vi "Get Publish Data Events.vi"(11 "UserEvents in":refnum<class "User Events.lvclass">) -> (2 "Publish Data Events":T1, 3 "UserEvents out":refnum<class "User Events.lvclass">)   [LabVIEW 2015, in "User Events.lvclass"]
uses:
  User Events.lvclass
  Typedefs/Publish Data Events.ctl
  Typedefs/State Types.ctl
  <userlib>/Common/ILC/Typedefs/Outputs.ctl
  <userlib>/Common/ILC/Typedefs/ADC Eng.ctl
  Typedefs/Scan Progress.ctl
  User Events.lvclass/User Events.ctl
  Typedefs/FAMT Typedefs.lvlib
  <userlib>/Common/ILC/Typedefs/ILCTypedefs.lvlib
panel:
  # "DAC"
  # "DAC"
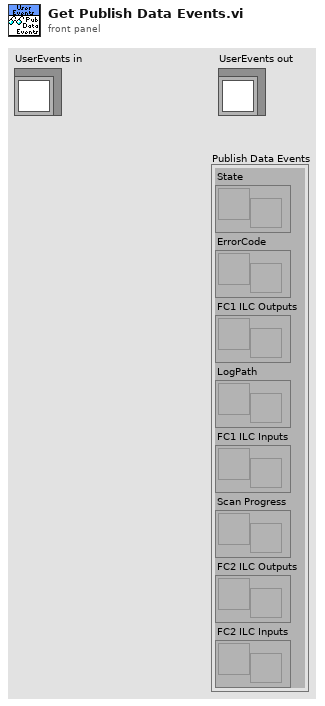
[diagram p1: front panel]
types:
  T1 = typedef "FAMT Typedefs.lvlib/Publish Data Events.ctl" = cluster{"State":refnum<user-event>, "ErrorCode":refnum<user-event>, "FC1 ILC Outputs":refnum<user-event>, "LogPath":refnum<user-event>, "FC1 ILC Inputs":refnum<user-event>, "Scan Progress":refnum<user-event>, "FC2 ILC Outputs":refnum<user-event>, "FC2 ILC Inputs":refnum<user-event>}
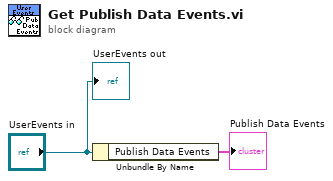
[diagram p0: block diagram]
diagram:
  n1 = Unbundle By Name("UserEvents in") -> ("Publish Data Events"=→"Publish Data Events":T1)
  "UserEvents out" <- "UserEvents in"
